vi "DEV INSERT.vi"() -> ()   [LabVIEW 2018, in "Database.lvlib"]
uses:
  Database.lvlib
  Items--cluster.ctl
  Purchased_Items--cluster.ctl
  Visits--cluster.ctl
panel:
  in  "Visits":T1 {"TotalSpend" format="£%.2g"; "SpendTaxedA" format="£%.2g"; "SpendTaxedB" format="£%.2g"}
  out "Output Data":string[][](array[string])
  out "Error Out":errorcluster
  out "resulting string":string
  in  "Purchased_Items":T2 {"TotalPriceIncludingDiscount" format="£%.2g"; "TotalDiscount" format="£%.2g"}
  in  "Items":T3
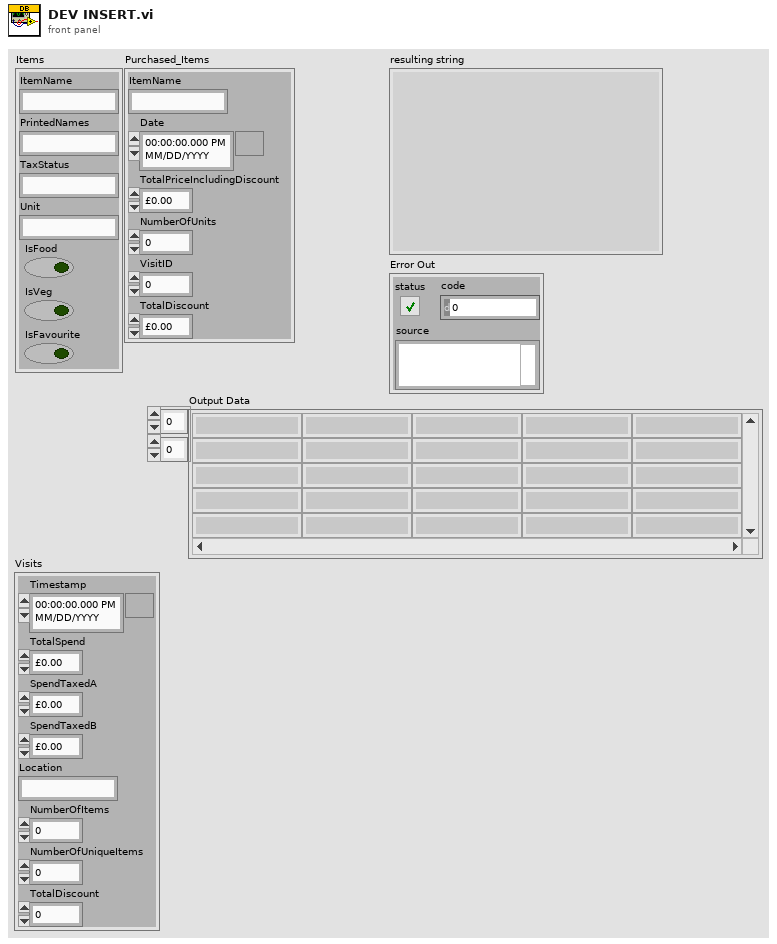
[diagram p1: front panel]
types:
  T1 = typedef "Database.lvlib/Visits--cluster.ctl" = cluster{"Timestamp":timestamp, "TotalSpend":dbl, "SpendTaxedA":dbl, "SpendTaxedB":dbl, "Location":string, "NumberOfItems":i32, "NumberOfUniqueItems":i32, "TotalDiscount":dbl}
  T2 = typedef "Database.lvlib/Purchased_Items--cluster.ctl" = cluster{"ItemName":string, "Date":timestamp, "TotalPriceIncludingDiscount":dbl, "NumberOfUnits":i32, "VisitID":i32, "TotalDiscount":dbl}
  T3 = typedef "Database.lvlib/Items--cluster.ctl" = cluster{"ItemName":string, "PrintedNames":string, "TaxStatus":string, "Unit":string, "IsFood":bool, "IsVeg":bool, "IsFavourite":bool}
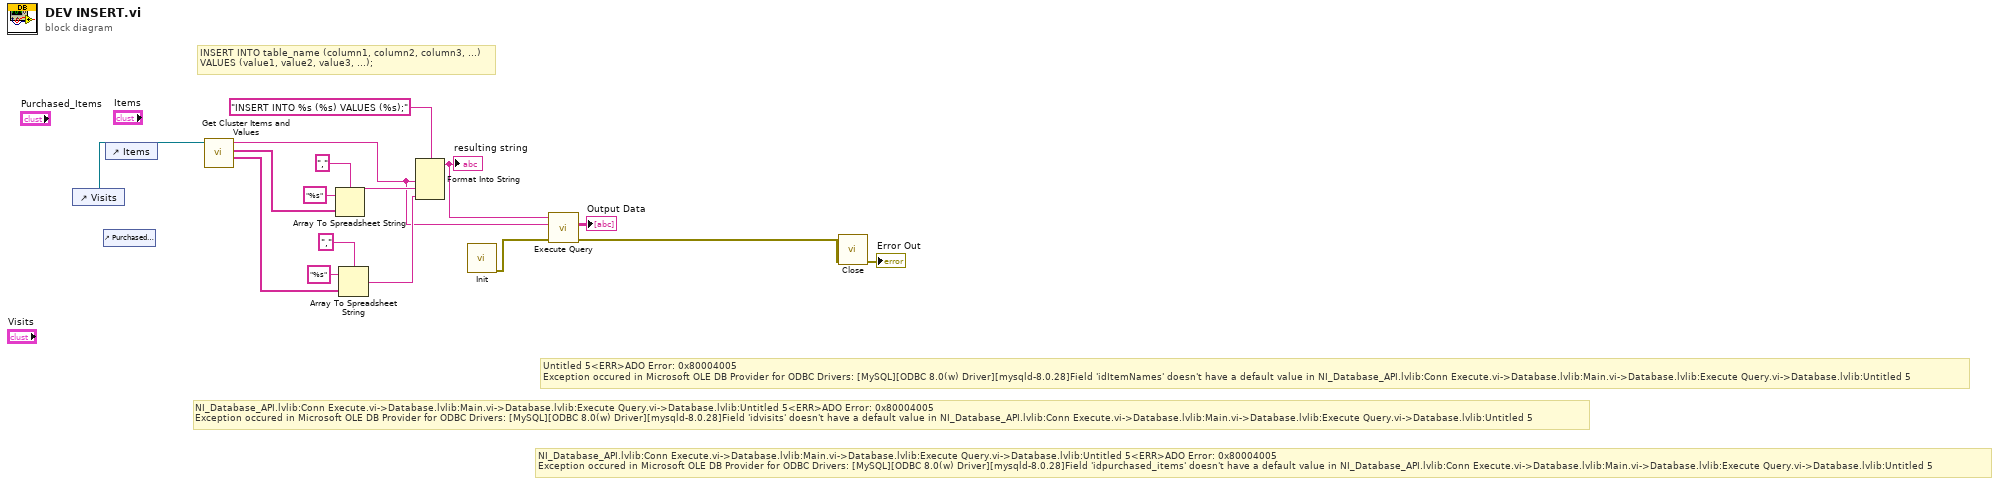
[diagram p0: block diagram]
diagram:
  # "NI_Database_API.lvlib:Conn Execute.vi->Database.lvlib:Main.vi->Database.lvlib:Execute Query.vi->Database.lvlib:Untitled 5<ERR>ADO Error: 0x80004005\nException occured in Microsoft OLE DB Provider for ODBC Drivers: [MySQL][ODBC 8.0(w) Driver][mysqld-8.0.28]Field 'idvisits' doesn't have a default value in NI_Database_API.lvlib:Conn Execute.vi->Database.lvlib:Main.vi->Database.lvlib:Execute Query.vi->Database.lvlib:Untitled 5"
  # "NI_Database_API.lvlib:Conn Execute.vi->Database.lvlib:Main.vi->Database.lvlib:Execute Query.vi->Database.lvlib:Untitled 5<ERR>ADO Error: 0x80004005\nException occured in Microsoft OLE DB Provider for ODBC Drivers: [MySQL][ODBC 8.0(w) Driver][mysqld-8.0.28]Field 'idpurchased_items' doesn't have a default value in NI_Database_API.lvlib:Conn Execute.vi->Database.lvlib:Main.vi->Database.lvlib:Execute Query.vi->Database.lvlib:Untitled 5"
  # "Untitled 5<ERR>ADO Error: 0x80004005\nException occured in Microsoft OLE DB Provider for ODBC Drivers: [MySQL][ODBC 8.0(w) Driver][mysqld-8.0.28]Field 'idItemNames' doesn't have a default value in NI_Database_API.lvlib:Conn Execute.vi->Database.lvlib:Main.vi->Database.lvlib:Execute Query.vi->Database.lvlib:Untitled 5"
  # "INSERT INTO table_name (column1, column2, column3, ...)\nVALUES (value1, value2, value3, ...);"
  n1 = control-ref of="Visits"() -> (w1:refnum<vi>)
  n2 = control-ref of="Purchased_Items"() -> ()  [unwired: 1 out]
  n3 = control-ref of="Items"() -> ()  [unwired: 1 out]
  n4 = call "Get Cluster Items and Values.vi"("Generic Cluster Reference"=w1) -> ("String Values"=w11:string[], "Column"=w14:string[], "Database"=w7:string)  [unwired: 7 in, 1 out]
  n5 = Array To Spreadsheet String(delimiter (Tab)=",", array=w14, 3:"%s" ("format string")) -> (spreadsheet string=w9:string)
  n6 = Array To Spreadsheet String(delimiter (Tab)=",", array=w11, 3:"%s" ("format string")) -> (spreadsheet string=w8:string)
  n7 = Format Into String(format string="INSERT INTO %s (%s) VALUES (%s);", w7, w9, w8) -> (resulting string=w6:string)  [unwired: 2 in, 1 out]
  "resulting string" <- w6
  n8 = call "Init.vi"() -> ("Error Out"=w5:errorcluster)  [unwired: 11 in]
  n9 = call "Execute Query.vi"("Error In"=w5, "Table"=w7, "Query"=w6) -> ("Error Out"=w4:errorcluster, "Output Data"=→"Output Data":string[][])  [unwired: 6 in, 1 out]
  n10 = call "Close.vi"("Error In"=w4) -> ("Error Out"=→"Error Out":errorcluster)  [unwired: 10 in]
